vi "Set BG Image.vi"(8 "error in (no error)":errorcluster, 11 "IMAQ Display in":refnum<class "HIJ IMAQdx Display.lvclass">) -> (0 "error out":errorcluster, 3 "IMAQ Display out":refnum<class "HIJ IMAQdx Display.lvclass">)   [LabVIEW 2014, in "HIJ IMAQdx Display.lvlib" / "HIJ IMAQdx Display.lvclass"]
uses:
  HIJ IMAQdx Display.lvclass
  HIJ Vision Display/HIJ Vision Display/HIJ Vision Display.lvclass/HIJ Vision Display.ctl
  HIJ IMAQdx Display.lvclass/HIJ IMAQdx Display.ctl
  HIJ Vision Display/HIJ Vision Display/HIJ Vision Display.lvclass
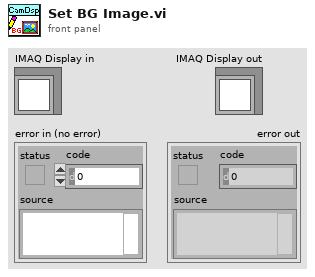
[diagram p1: front panel]
types:
  T1 = typedef "IMAQ Image.ctl" = refnum<image>
  T2 = typedef "Image Type" = u32
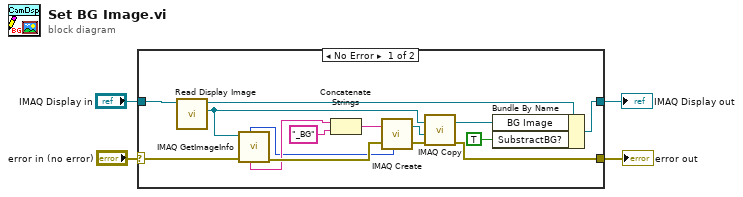
[diagram p0: block diagram]
diagram:
  n1 = case shown="No Error" "error in (no error)" {
    selector: "error in (no error)" -> [w6 w20]
    tunnel: [w5 w20] -> w3
    tunnel: [w19 w21] -> w1
    tunnel: "IMAQ Display in" -> [w10 w21]
    frame No Error {
      n2 = call "Read Display Image.vi"("HIJ Vision Display in"=w10) -> ("Image"=w7:T1, "HIJ Vision Display out"=w8:refnum<class "HIJ IMAQdx Display.lvclass">)  [unwired: 9 in]
      n3 = call "IMAQ GetImageInfo"("error in (no error)"=w6, "Image"=w7) -> ("error out"=w16:errorcluster, "Image Name"=w12:string, "Image Type"=w11:T2)  [unwired: 2 in, 5 out]
      n4 = Concatenate Strings(w12, "_BG" ("string")) -> (w13:string)
      n5 = call "IMAQ Create"("Image Name"=w13, "Image Type"=w11, "error in (no error)"=w16) -> ("New Image"=w15:T1, "error out"=w17:errorcluster)  [unwired: 2 in]
      n6 = call "IMAQ Copy"("error in (no error)"=w17, "Image Dst"=w15, "Image Src"=w7) -> ("error out"=w5:errorcluster, "Image Dst Out"=w9:T1)  [unwired: 3 in]
      n7 = Bundle By Name(cluster=w8, "BG Image"=w9, "SubstractBG?"=TRUE) -> (w19:refnum<class "HIJ IMAQdx Display.lvclass">)
    }
    frame Error {
    }
  }
  "error out" <- w3
  "IMAQ Display out" <- w1
